vi "DSF.Engine.Builder.Set Builder Status.vi"(10 "Builder Status":refnum<class "Builder Status.lvclass">, 11 "Builder in":refnum<class "DSF.Engine.Builder.lvclass">) -> (3 "Builder out":refnum<class "DSF.Engine.Builder.lvclass">)   [LabVIEW 2016, in "DSF.Engine.lvlib" / "DSF.Engine.Builder.lvclass"]
uses:
  DSF.Engine.Builder.lvclass
  Status/Builder Status.lvclass
  DSF.Engine.Builder.lvclass/DSF.Engine.Builder.ctl
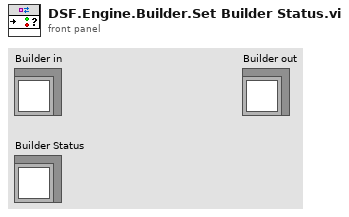
[diagram p1: front panel]
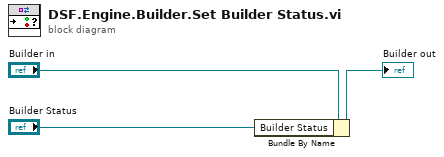
[diagram p0: block diagram]
diagram:
  n1 = Bundle By Name(cluster="Builder in", "Builder Status"="Builder Status") -> (→"Builder out":refnum<class "DSF.Engine.Builder.lvclass">)
